vi "ExSubInitSimpleNoStore.vi"(2 "Intensifier":bool, 3 "Shutter Comp":cluster{"Open in ms":u32, "Close in ms":u32}={"Open in ms"=8, "Close in ms"=8}, 4 "error in (no error)":errorcluster, 5 "Triggering mode":u32, 6 "Exposure":dbl min=0.0 step=1e-06 format="%.5f", 7 "Camera Handle":u32) -> (0 "error out":errorcluster, 1 "Handles":cluster{"Camera":u32, "File":u32, "Image":u32})   [LabVIEW 2010]
panel:
  # "ExSubInitSimple: this does the basic initializations"
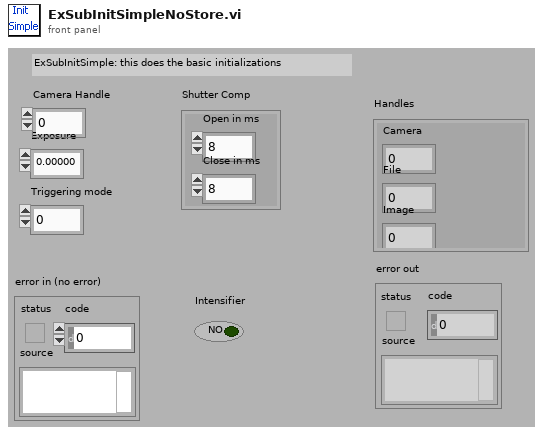
[diagram p1: front panel]
types:
  T1 = cluster{"Camera Handle":u32, "File Handle":u32, "Image Handle":u32}
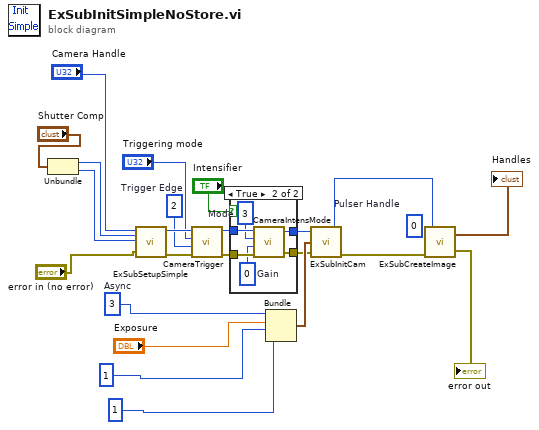
[diagram p0: block diagram]
diagram:
  w11 = 3  # Async
  (unwired) u32 0  # Pulser Handle
  w18 = u32 2  # Trigger Edge
  n1 = Unbundle("Shutter Comp") -> ("Open in ms"=w2:u32, "Close in ms"=w1:u32)
  n2 = call "ExSubSetupSimple.vi"("error in (no error)"="error in (no error)", "Close comp time"=w1, "Open comp time"=w2, "Camera Handle"="Camera Handle") -> ("error out"=w19:errorcluster, "Camera Handle"=w20:u32)
  n3 = call <userlib>:"CameraTrigger.vi"("error in"=w19, "Trigger Edge"=w18, "Timing Mode"="Triggering mode", "Camera Handle"=w20) -> ("error out"=w14:errorcluster, "Camera Handle"=w16:u32)
  n4 = case shown="True" "Intensifier" {
    tunnel: w16 -> [w25 w31]
    tunnel: [w25 w30] -> w15
    tunnel: w14 -> [w24 w29]
    tunnel: [w24 w28] -> w13
    frame False {
    }
    frame True {
      w26 = u32 0  # Gain
      w27 = u32 3  # Mode
      n5 = call <userlib>:"CameraIntensMode.vi"("error in"=w29, "Intensifier Gain"=w26, "Mode"=w27, "Camera Handle"=w31) -> ("error out"=w28:errorcluster, "Camera Handle"=w30:u32)
    }
  }
  n6 = Bundle("Async"=w11, "Exposure"="Exposure", 1, 1) -> (w22:cluster{"Async":i32, "Exposure":dbl, i32, i32})  [unwired: 1 in]
  n7 = call "ExSubInitCam.vi"("error in (no error)"=w13, "Camera Information"=w22, "Camera Handle"=w15) -> ("error out"=w21:errorcluster, "Camera Handle"=w17:u32)
  n8 = call "ExSubCreateImage.vi"("error in (no error)"=w21, "Camera Handle"=w17) -> ("error out"=→"error out":errorcluster, "Handles Out"=→"Handles":T1)  [unwired: 2 in]
